vi "NUM TO 1D LED(SubVI).vi"(1 "A":dbl) -> (0 "Array":bool[](array[boolean]))   [LabVIEW 2019]
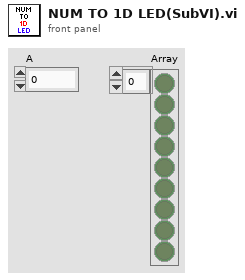
[diagram p1: front panel]
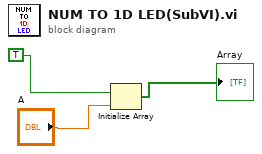
[diagram p0: block diagram]
diagram:
  n1 = Initialize Array "Initialize Array"(TRUE, "A") -> (→"Array":bool[])
